vi "to string.vi"(8 "error in":errorcluster, 11 "configuration in":refnum<class "Device Configuration.lvclass">) -> (0 "error out":errorcluster, 1 "data":string, 2 "version":string, 3 "configuration out":refnum<class "Device Configuration.lvclass">)   [LabVIEW 2014, in "Device Configuration.lvclass"]
doc: "Provides an interface for saving a module configuration to a file or other serialized data source. It is recommended that all children of this class store data in two sets--data required for its own initialization, and any data required for parent initialization--and that each implementation uses the <b>Call Parent Method</b> primitive to serialize parent information."
uses:
  Device Configuration.lvclass
  Device Configuration.lvclass/Device Configuration.ctl
  <vilib>/NI/Configuration Framework/serializable configuration/NISE_CEF_serializable configuration.lvclass
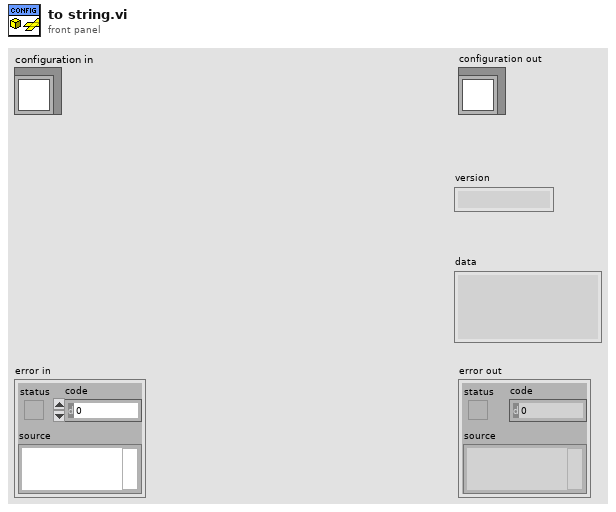
[diagram p1: front panel]
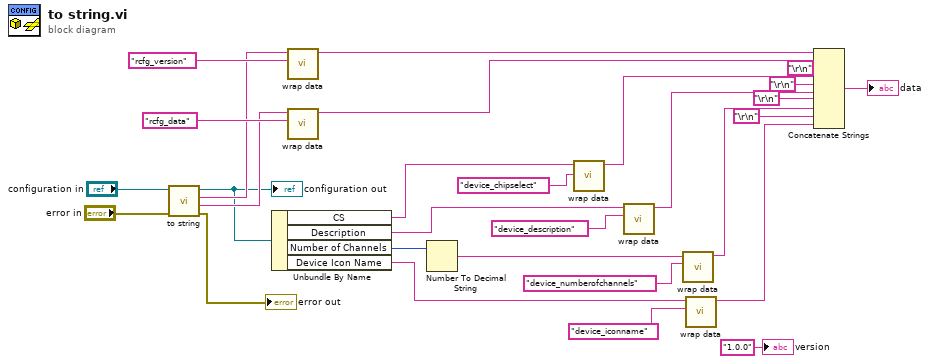
[diagram p0: block diagram]
diagram:
  n1 = call-parent "to string.vi"("error in"="error in", "configuration in"="configuration in") -> ("error out"=→"error out":errorcluster, "data"=w21:string, "version"=w22:string, "configuration out"=w6:refnum<class "Device Configuration.lvclass">)  [unwired: 6 in]
  "configuration out" <- w6
  n2 = Unbundle By Name(w6) -> ("CS"=w12:string, "Description"=w11:string, "Number of Channels"=w10:u32, "Device Icon Name"=w1:string)
  n3 = call <vilib>:"wrap data.vi"("identifier"="rcfg_version", "data to wrap"=w22) -> ("wrapped data"=w26:string)  [unwired: 9 in]
  n4 = call <vilib>:"wrap data.vi"("identifier"="rcfg_data", "data to wrap"=w21) -> ("wrapped data"=w25:string)  [unwired: 9 in]
  n5 = Number To Decimal String(number=w10) -> (decimal integer string=w9:string)  [unwired: 1 in]
  n6 = call <vilib>:"wrap data.vi"("identifier"="device_chipselect", "data to wrap"=w12) -> ("wrapped data"=w23:string)  [unwired: 9 in]
  n7 = call <vilib>:"wrap data.vi"("identifier"="device_description", "data to wrap"=w11) -> ("wrapped data"=w16:string)  [unwired: 9 in]
  n8 = call <vilib>:"wrap data.vi"("identifier"="device_numberofchannels", "data to wrap"=w9) -> ("wrapped data"=w4:string)  [unwired: 9 in]
  n9 = call <vilib>:"wrap data.vi"("identifier"="device_iconname", "data to wrap"=w1) -> ("wrapped data"=w2:string)  [unwired: 9 in]
  n10 = Concatenate Strings(w26, w25, "\r\n", w23, "\r\n", w16, "\r\n", w4, "\r\n", w2) -> (→"data":string)
  "version" <- "1.0.0" ("version")
